vi "StateSpaceUtil_Check_Stabilizable.vi"(9 "B":T1, 11 "A":T1) -> (0 "Error":bool, 3 "IsStabilizable":bool, 4 "Eigenvalues":cdb[](array[numeric]), 6 "R rank":i32[](array[numeric]))   [LabVIEW 2019, in "Trajectory_Library.lvlib"]
doc: "THIS IS AN INTERNAL ROUTINE. USE IsStabalizable INSTEAD.\nReturns true if (A, B) is a stabilizable pair.\n \n(A,B) is stabilizable if and only if the uncontrollable eigenvalues of A, if any, have absolute values less than one, where an eigenvalue is uncontrollable if rank(Lambda - A, B) < n where n is number of states.\n \nInputs:\n - A -- System matrix.\n - B -- nput matrix.\n\nOutputs:\n - IsStablizable -- If the system is stabilizable."
uses:
  <vilib>/Analysis/Matrix/Datatypes/RealMatrix.ctl
  <vilib>/Analysis/7linalg.llb/Eigenvalue and Vectors Output Option.ctl
  <vilib>/Analysis/7linalg.llb/Complex QR Decomposition.vi
  <vilib>/Analysis/_algsub.llb/Complex Matrix Rank.vi
  <vilib>/Analysis/Matrix/Numeric/Conversions/Array To Matrix - CA2.vi
  <vilib>/Analysis/7linalg.llb/Real Eigenvalues and Vectors.vi
  <vilib>/Analysis/7linalg.llb/Create Special Complex Matrix.vi
  <vilib>/Analysis/Matrix/Numeric/Multiply/Multiply - CM,C.vi
  <vilib>/Analysis/Matrix/Numeric/Subtract/Subtract - CM,CM.vi
  Trajectory_Library.lvlib
  <vilib>/Analysis/NI_AALPro.lvlib
  <vilib>/Analysis/Matrix/NI_Matrix.lvlib
panel:
  # "<States, States>"
  # "<States, Inputs>"
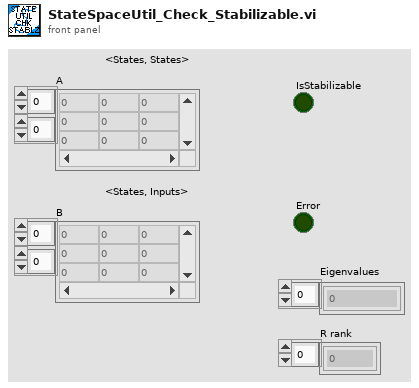
[diagram p1: front panel]
types:
  T1 = typedef "NI_Matrix.lvlib/RealMatrix.ctl" = dbl[][]
  T2 = typedef "NI_AALPro.lvlib/Eigenvalue and Vectors Output Option.ctl" = i32
  T3 = typedef "NI_Matrix.lvlib/ComplexMatrix.ctl" = cdb[][]
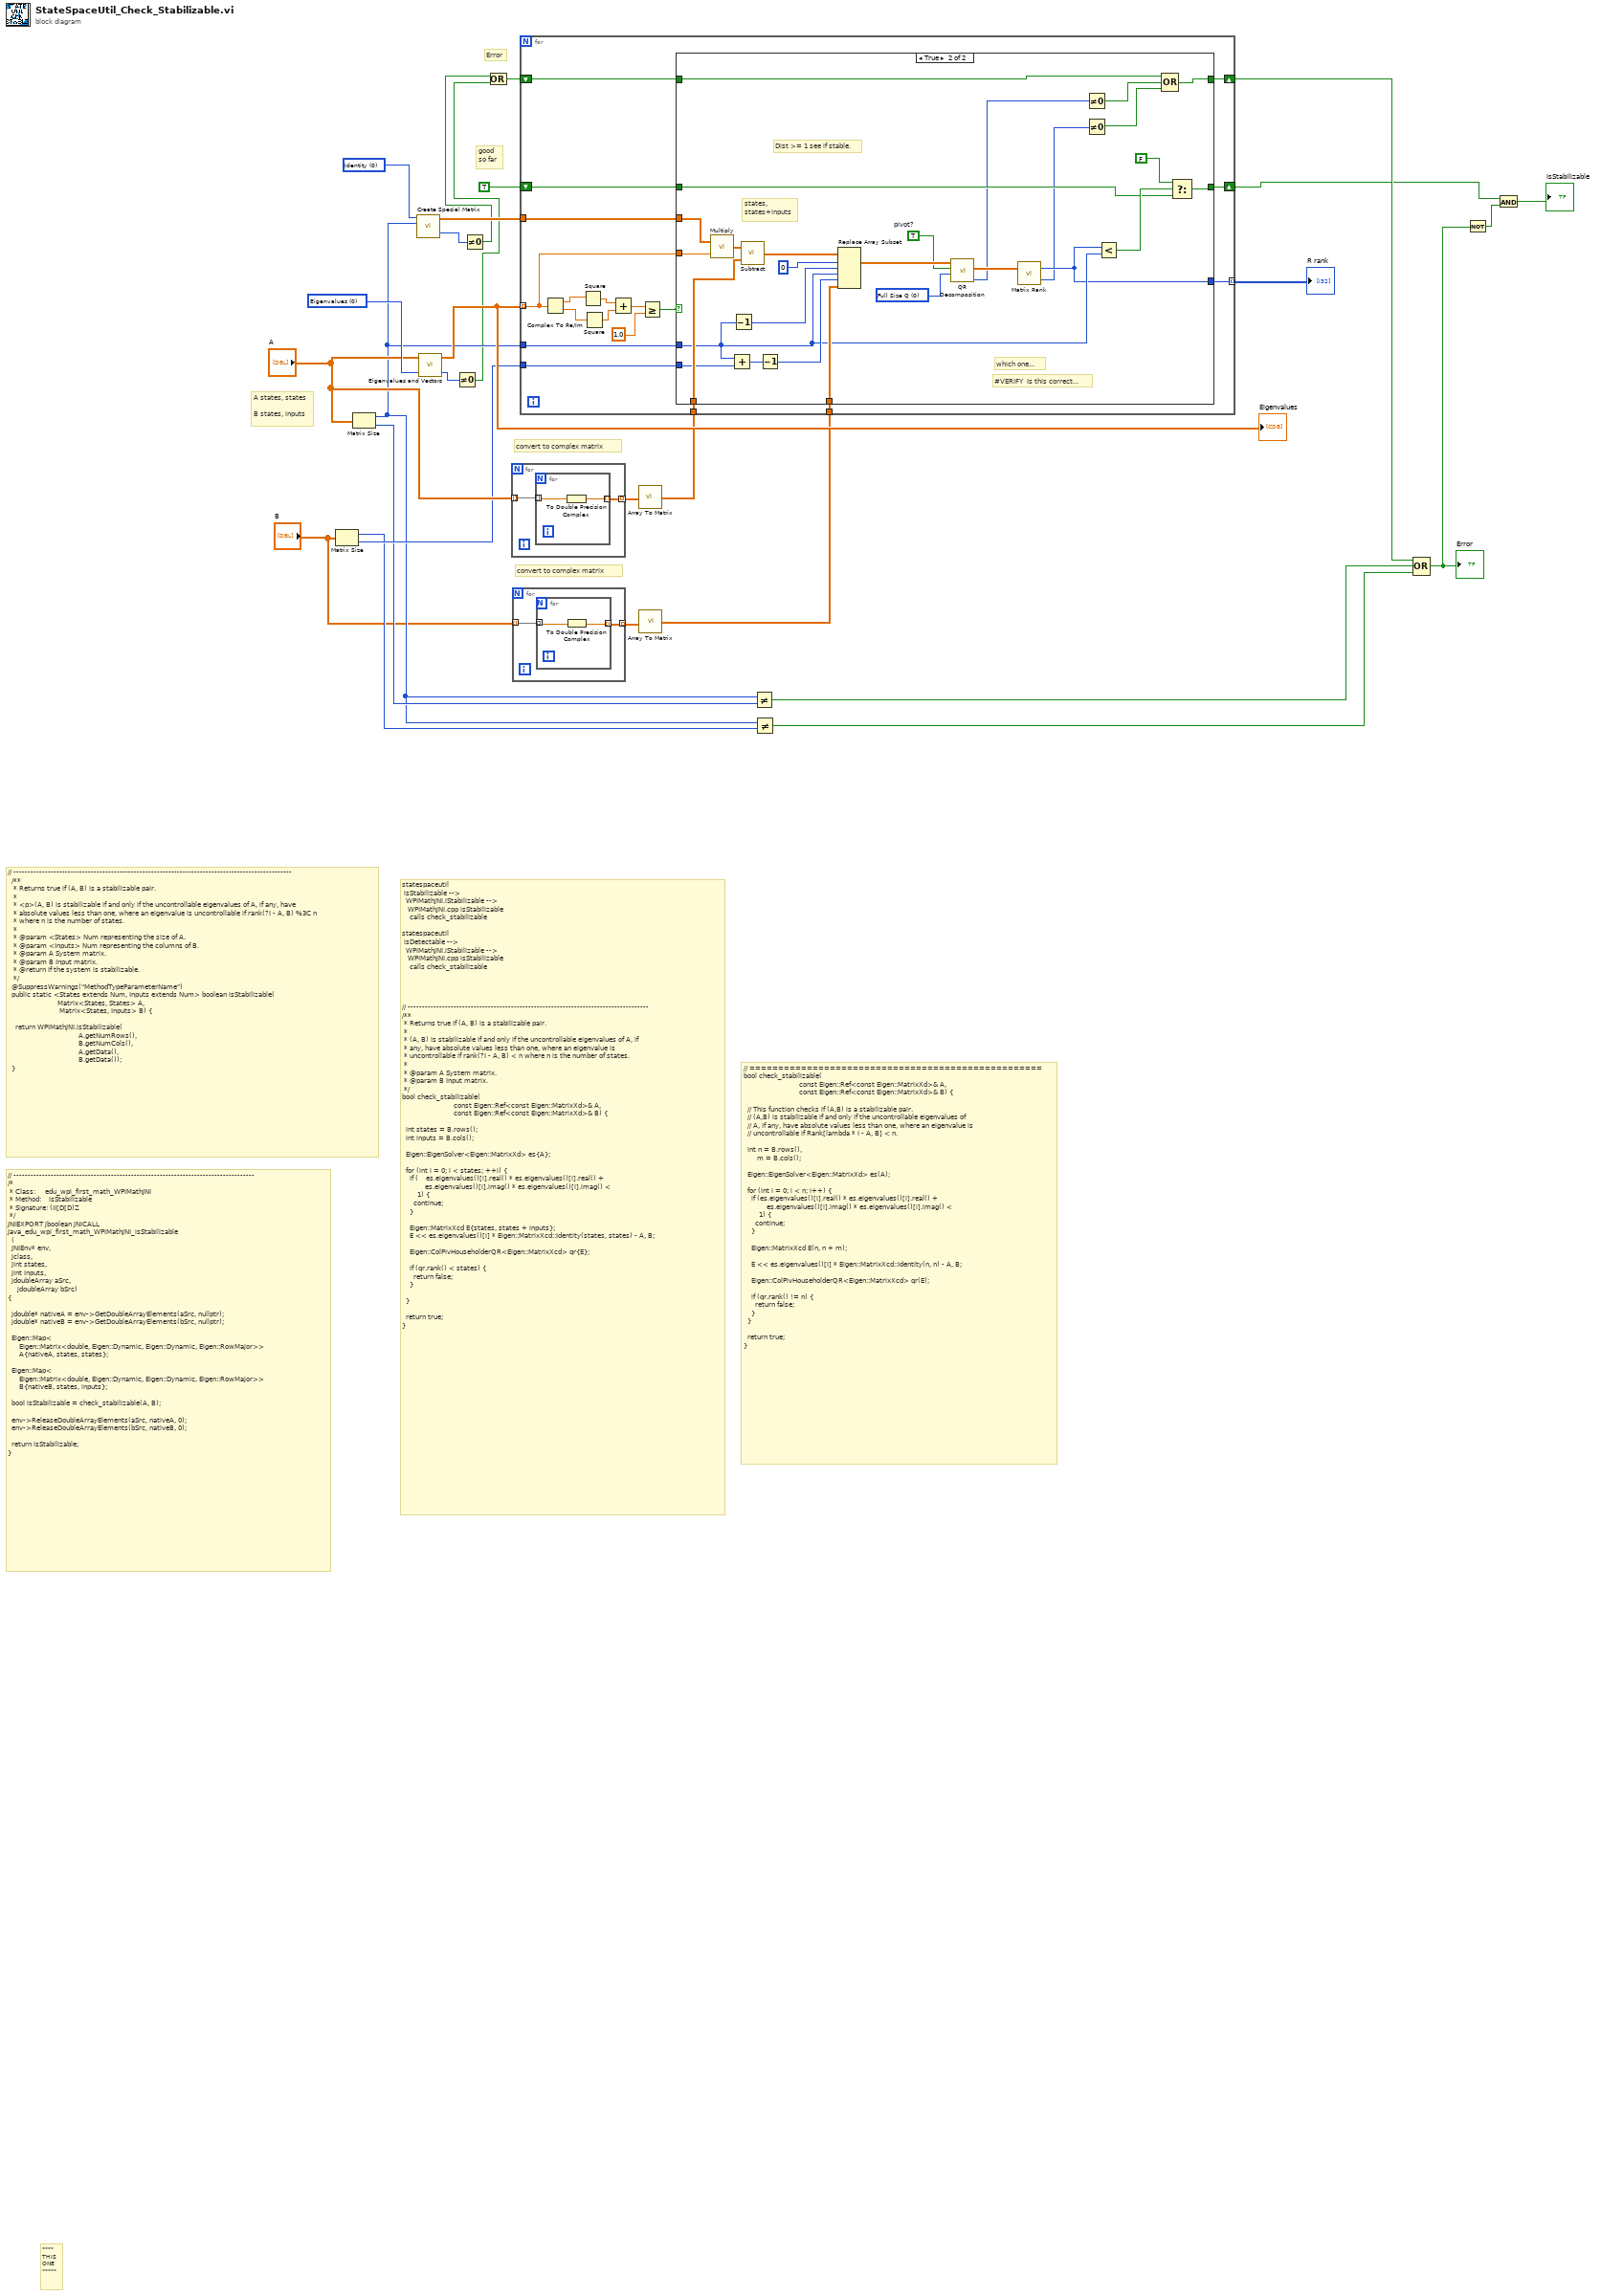
[diagram p0: block diagram]
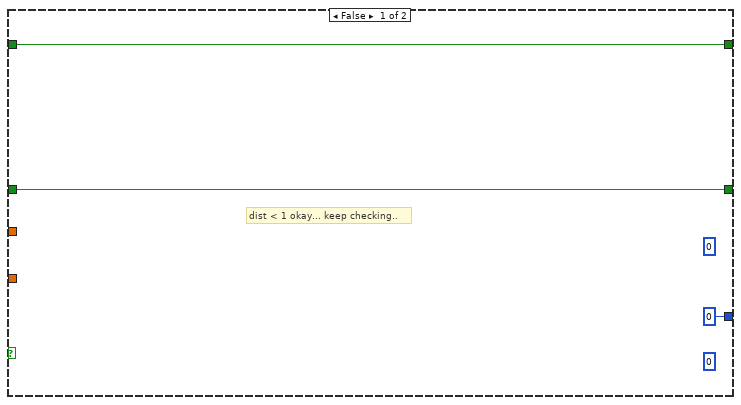
[diagram p2: hidden frame]
diagram:
  w24 = 0 items=["Identity", "Diagonal", "Toeplitz", "Vandermonde", "Companion", "Hankel", "Hadamard", "Wilkinson", "Hilbert", "Inverse Hilbert", "Rosser", "Pascal"] ("matrix type")
  w28 = T2 0 items=["Eigenvalues", "Eigenvalues & Vectors"] ("output option")
  # "Error"
  # "convert to complex matrix"
  # "convert to complex matrix"
  # "good \nso far"
  # "A states, states\n\nB states, inputs"
  # "// ------------------------------------------------------------------------------------\n/*\n * Class:     edu_wpi_first_math_WPIMathJNI\n * Method:    isStabilizable\n * Signature: (II[D[D)Z\n */\nJNIEXPORT jboolean JNICALL\nJava_edu_wpi_first_math_WPIMathJNI_isStabilizable\n  (\n\t\tJNIEnv* env, \n\t\tjclass, \n\t\tjint states, \n\t\tjint inputs, \n\t\tjdoubleArray aSrc,\n   \t\tjdoubleArray bSrc)\n{\n\n  jdouble* nativeA = env->GetDoubleArrayElements(aSrc, nullptr);\n  jdouble* nativeB = env->GetDoubleArrayElements(bSrc, nullptr);\n\n  Eigen::Map<\n      Eigen::Matrix<double, Eigen::Dynamic, Eigen::Dynamic, Eigen::RowMajor>>\n      A{nativeA, states, states};\n\n  Eigen::Map<\n      Eigen::Matrix<double, Eigen::Dynamic, Eigen::Dynamic, Eigen::RowMajor>>\n      B{nativeB, states, inputs};\n\n  bool isStabilizable = check_stabilizable(A, B);\n\n  env->ReleaseDoubleArrayElements(aSrc, nativeA, 0);\n  env->ReleaseDoubleArrayElements(bSrc, nativeB, 0);\n\n  return isStabilizable;\n}"
  # "statespaceutil\n\tisStabilizable --> \n\t\tWPIMathJNI.iStabilizable --> \n\t\t\tWPIMathJNI.cpp isStabilizable  \n\t\t\t\tcalls check_stabilizable\n\nstatespaceutil\n\tisDetectable -->  \n\t\tWPIMathJNI.iStabilizable --> \n\t\t\tWPIMathJNI.cpp isStabilizable\n\t\t\t\tcalls check_stabilizable\n\n\n\n\n// ------------------------------------------------------------------------------------\n/**\n * Returns true if (A, B) is a stabilizable pair.\n *\n * (A, B) is stabilizable if and only if the uncontrollable eigenvalues of A, if\n * any, have absolute values less than one, where an eigenvalue is\n * uncontrollable if rank(?I - A, B) < n where n is the number of states.\n *\n * @param A System matrix.\n * @param B Input matrix.\n */\nbool check_stabilizable(\n                           const Eigen::Ref<const Eigen::MatrixXd>& A,\n                           const Eigen::Ref<const Eigen::MatrixXd>& B) {\n\n  int states = B.rows();\n  int inputs = B.cols();\n\n  Eigen::EigenSolver<Eigen::MatrixXd> es{A};\n\n  for (int i = 0; i < states; ++i) {\n    if (    es.eigenvalues()[i].real() * es.eigenvalues()[i].real() +\n            es.eigenvalues()[i].imag() * es.eigenvalues()[i].imag() <\n        1) {\n      continue;\n    }\n\n    Eigen::MatrixXcd E{states, states + inputs};\n    E << es.eigenvalues()[i] * Eigen::MatrixXcd::Identity(states, states) - A, B;\n\n    Eigen::ColPivHouseholderQR<Eigen::MatrixXcd> qr{E};\n\n    if (qr.rank() < states) {\n      return false;\n    }\n\n  }\n\n  return true;\n}"
  # "// ===================================================\nbool check_stabilizable(\n                             const Eigen::Ref<const Eigen::MatrixXd>& A,\n                             const Eigen::Ref<const Eigen::MatrixXd>& B) {\n\n  // This function checks if (A,B) is a stabilizable pair.\n  // (A,B) is stabilizable if and only if the uncontrollable eigenvalues of\n  // A, if any, have absolute values less than one, where an eigenvalue is\n  // uncontrollable if Rank[lambda * I - A, B] < n.\n\n  int n = B.rows(), \n       m = B.cols();\n\n  Eigen::EigenSolver<Eigen::MatrixXd> es(A);\n\n  for (int i = 0; i < n; i++) {\n    if (es.eigenvalues()[i].real() * es.eigenvalues()[i].real() +\n            es.eigenvalues()[i].imag() * es.eigenvalues()[i].imag() <\n        1) {\n      continue;\n    }\n\n    Eigen::MatrixXcd E(n, n + m);\n\n    E << es.eigenvalues()[i] * Eigen::MatrixXcd::Identity(n, n) - A, B;\n\n    Eigen::ColPivHouseholderQR<Eigen::MatrixXcd> qr(E);\n\n    if (qr.rank() != n) {\n      return false;\n    }\n  }\n\n  return true;\n}"
  # "// -------------------------------------------------------------------------------------------------\n  /**\n   * Returns true if (A, B) is a stabilizable pair.\n   *\n   * <p>(A, B) is stabilizable if and only if the uncontrollable eigenvalues of A, if any, have\n   * absolute values less than one, where an eigenvalue is uncontrollable if rank(?I - A, B) %3C n\n   * where n is the number of states.\n   *\n   * @param <States> Num representing the size of A.\n   * @param <Inputs> Num representing the columns of B.\n   * @param A System matrix.\n   * @param B Input matrix.\n   * @return If the system is stabilizable.\n   */\n  @SuppressWarnings(\"MethodTypeParameterName\")\n  public static <States extends Num, Inputs extends Num> boolean isStabilizable(\n                          Matrix<States, States> A, \n                           Matrix<States, Inputs> B) {\n\n    return WPIMathJNI.isStabilizable(\n                                   \t\tA.getNumRows(), \n                                   \t\tB.getNumCols(), \n                                   \t\tA.getData(), \n                                   \t\tB.getData());\n  }"
  # "****\nTHIS\nONE\n*****"
  n1 = Matrix Size(0:"B") -> (1:w17:i32, 2:w20:i32)
  n2 = Matrix Size(0:"A") -> (1:w18:i32, 2:w19:i32)
  n3 = call-poly <vilib>:"Create Special Matrix.vi"("matrix type"=w24, "matrix size"=w18) -> ("Special Matrix"=w25:T3, "error"=w12:i32)  [unwired: 3 in]
  n4 = call-poly <vilib>:"Eigenvalues and Vectors.vi"("output option"=w28, "Input Matrix"="A") -> ("error"=w13:i32, "Eigenvalues"=w27:cdb[])  [unwired: 1 in, 1 out]
  "Eigenvalues" <- w27
  n5 = Not Equal To 0?(x=w13) -> (x != 0?=w9:bool)
  n6 = Not Equal To 0?(x=w12) -> (x != 0?=w10:bool)
  n7 = Or(x=w10, y=w9) -> (x .or. y?=w11:bool)
  n8 = for {
    tunnel: "A" -> [w30] mode=indexing
    tunnel: [w29] -> w22 mode=indexing
    n9 = for {
      tunnel: w30 -> [w32] mode=indexing
      tunnel: [w31] -> w29 mode=indexing
      n10 = To Double Precision Complex(1:w32) -> (0:w31:cdb)
    }
  }
  n11 = for {
    tunnel: "B" -> [w34] mode=indexing
    tunnel: [w33] -> w16 mode=indexing
    n12 = for {
      tunnel: w34 -> [w36] mode=indexing
      tunnel: [w35] -> w33 mode=indexing
      n13 = To Double Precision Complex(1:w36) -> (0:w35:cdb)
    }
  }
  n14 = call-poly <vilib>:"Array To Matrix.vi"("Complex 2D Array"=w22) -> ("Complex Matrix"=w21:T3)
  n15 = call-poly <vilib>:"Array To Matrix.vi"("Complex 2D Array"=w16) -> ("Complex Matrix"=w14:T3)
  n16 = for {
    tunnel: w27 -> [w45] mode=indexing
    shift-right: [w40] -> w5
    shift-left: TRUE -> [w47]
    tunnel: w25 -> [w46]
    tunnel: w21 -> [w44]
    tunnel: w20 -> [w43]
    tunnel: w18 -> [w42]
    tunnel: w14 -> [w41]
    shift-right: [w39] -> w6
    shift-left: w11 -> [w38]
    tunnel: [w37] -> w1 mode=indexing
    n17 = Complex To Re/Im(x + iy=w45) -> (x=w54:dbl, y=w53:dbl)
    n18 = Square(x=w54) -> (x^2=w52:dbl)
    n19 = Square(x=w53) -> (x^2=w51:dbl)
    n20 = Add(x=w52, y=w51) -> (x+y=w50:dbl)
    n21 = Greater Or Equal?(x=w50, y=1.0) -> (x >= y?=w48:bool)
    n22 = case shown="True" w48 {
      tunnel: w47 -> [w57 w68]
      tunnel: [w57 w67] -> w40
      tunnel: w46 -> [_ w82]
      tunnel: w45 -> [_ w83]
      tunnel: w44 -> [_ w81]
      tunnel: w43 -> [_ w80]
      tunnel: w42 -> [_ w70]
      tunnel: w41 -> [_ w74]
      tunnel: [w56 w65] -> w39
      tunnel: w38 -> [w56 w64]
      tunnel: [0 ("rank") w59] -> w37
      frame False {
        (unwired) 0 ("rank")
        (unwired) 0 ("rank")
        # "dist < 1 okay... keep checking.."
      }
      frame True {
        w71 = u16 0 items=["Full Size Q", "Economy Size Q", "No Q"] ("Q option")
        w72 = TRUE  # pivot?
        # "#VERIFY  Is this correct..."
        # "which one..."
        # "states, \nstates+inputs"
        # "Dist >= 1 see if stable."
        n23 = call-poly <vilib>:"Multiply.vi"("Complex Scalar c"=w83, "Complex Matrix A"=w82) -> ("A * c"=w84:T3)
        n24 = Add(x=w70, y=w80) -> (x+y=w76:i32)
        n25 = Decrement(x=w70) -> (x-1=w77:i32)
        n26 = call-poly <vilib>:"Subtract.vi"("Complex Matrix B"=w81, "Complex Matrix A"=w84) -> ("A - B"=w79:T3)
        n27 = Decrement(x=w76) -> (x-1=w75:i32)
        n28 = Replace Array Subset(array=w79, new element=w74, index (dim 0)=0 ("row 1"), index (dim 1)=w77, index (dim 2)=w70, index (dim 3)=w75) -> (w73:T3)
        n29 = call-poly <vilib>:"QR Decomposition.vi"("Q option"=w71, "pivot?"=w72, "A"=w73) -> ("error"=w61:i32, "R"=w63:T3)  [unwired: 5 in, 2 out]
        n30 = call-poly <vilib>:"Matrix Rank.vi"("Input Matrix"=w63) -> ("error"=w58:i32, "rank"=w59:i32)  [unwired: 1 in]
        n31 = Not Equal To 0?(x=w61) -> (x != 0?=w62:bool)
        n32 = Not Equal To 0?(x=w58) -> (x != 0?=w60:bool)
        n33 = Less?(x=w59, y=w70) -> (x < y?=w69:bool)
        n34 = Compound Arithmetic op=OR(w64, w62, w60) -> (w65:bool)
        n35 = Select(t=FALSE, s=w69, f=w68) -> (s? t:f=w67:bool)
      }
    }
  }
  "R rank" <- w1
  n36 = Not Equal?(x=w18, y=w19) -> (x != y?=w7:bool)
  n37 = Not Equal?(x=w18, y=w17) -> (x != y?=w8:bool)
  n38 = Compound Arithmetic op=OR(w6, w7, w8) -> (w2:bool)
  "Error" <- w2
  n39 = Not(x=w2) -> (.not. x?=w4:bool)
  n40 = And(x=w5, y=w4) -> (x .and. y?=→"IsStabilizable":bool)
